vi "VISA MP-285 Get Position Improved Version v070925.vi"(0 "Input: Duty Cluster":T1) -> (1 "Output: X axis (microns)":dbl format="%.2f", 2 "Output: Y axis (microns)":dbl format="%.2f", 3 "Output: Z axis (microns)":dbl format="%.2f", 4 "Output: Duty Cluster":T1)   [LabVIEW 2010]
panel:
  out "Boolean":bool
  out "Serial Read":string
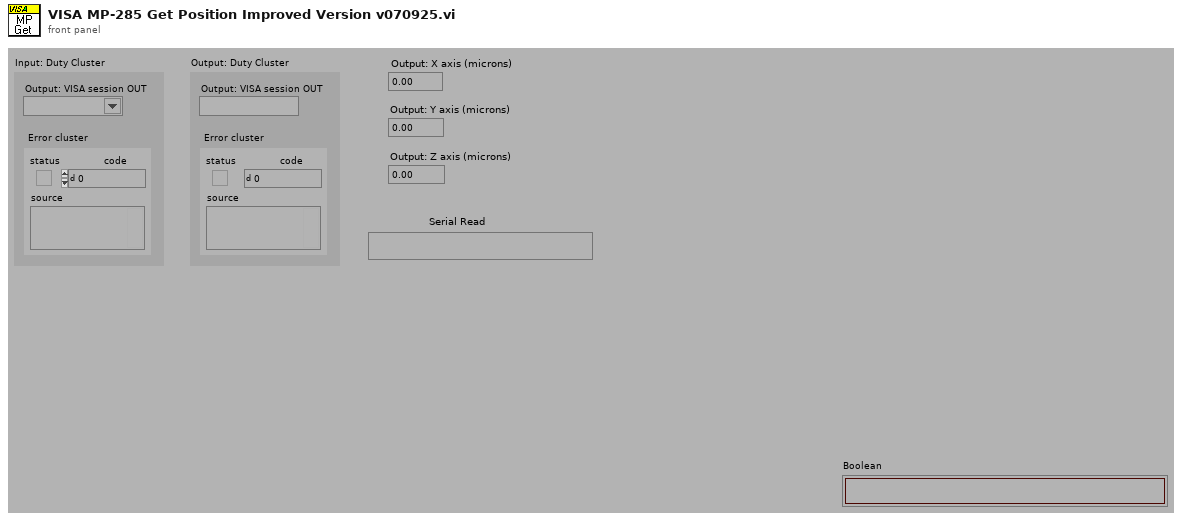
[diagram p1: front panel]
types:
  T1 = cluster{"Output: VISA session OUT":refnum<visa-resource-name>, "Error cluster":errorcluster}
  T2 = cluster{"Output: VISA session OUT":refnum<visa-resource-name>, "error out":errorcluster}
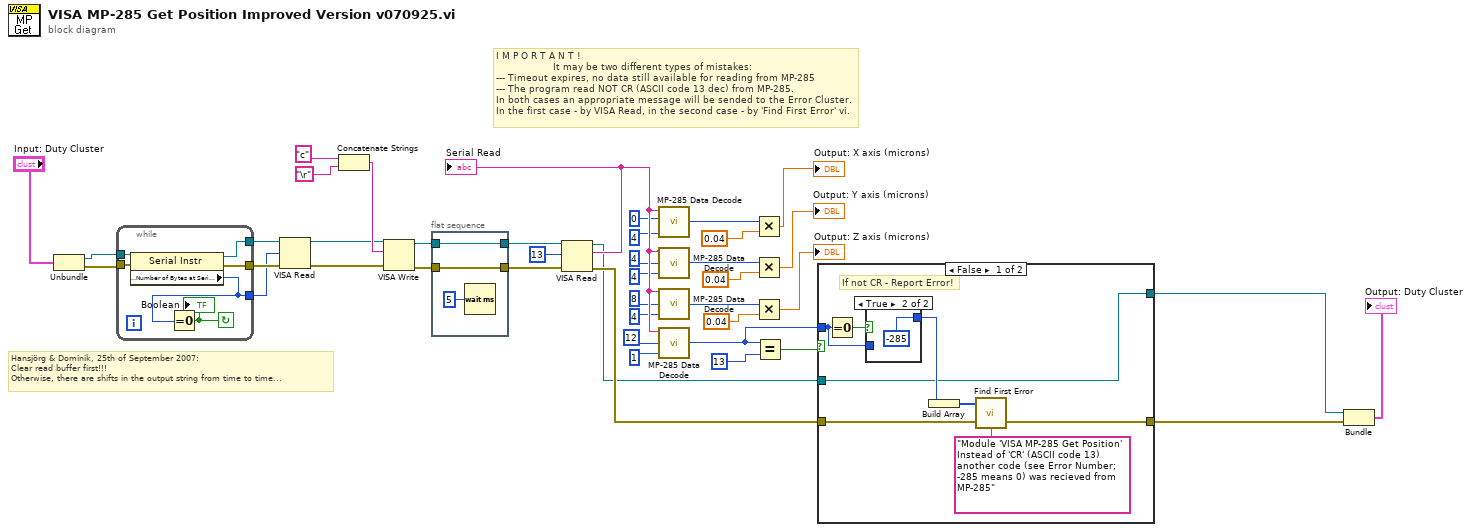
[diagram p0: block diagram]
diagram:
  # "Hansjörg & Dominik, 25th of September 2007: \nClear read buffer first!!!\nOtherwise, there are shifts in the output string from time to time..."
  # "I M P O R T A N T !\n                   It may be two different types of mistakes: \n--- Timeout expires, no data still available for reading from MP-285\n--- The program read NOT CR (ASCII code 13 dec) from MP-285.\nIn both cases an appropriate message will be sended to the Error Cluster.\nIn the first case - by VISA Read, in the second case - by 'Find First Error' vi."
  n1 = Unbundle("Input: Duty Cluster") -> ("Output: VISA session OUT"=w4:refnum<visa-resource-name>, "Error cluster"=w3:errorcluster)
  n2 = while {
    tunnel: [w45] -> w5
    tunnel: [w46] -> w6
    tunnel: [w47] -> w7
    tunnel: w3 -> [w48]
    tunnel: w4 -> [w43]
    stop <- w44 continue-if-true
    n3 = property class="Serial Instr"(reference=w43, error in=w48) -> (reference out=w46:refnum<visa-resource-name>, error out=w47:errorcluster, "Serial Settings:Number of Bytes at Serial Port"=w45:u32)
    n4 = Equal To 0?(x=w45) -> (x = 0?=w44:bool)
    "Boolean" <- w44
  }
  n5 = VISA Read(VISA resource name=w6, byte count=w5, error in (no error)=w7) -> (VISA resource name out=w2:refnum<visa-resource-name>, error out=w1:errorcluster)  [unwired: 2 out]
  n6 = Concatenate Strings("c", "\r") -> (w33:string)
  n7 = VISA Write(VISA resource name=w2, write buffer=w33, error in (no error)=w1) -> (VISA resource name out=w13:refnum<visa-resource-name>, error out=w11:errorcluster)  [unwired: 1 out]
  n8 = flat-sequence {
    tunnel: w13 -> [w51]
    tunnel: [w51] -> w12
    tunnel: w11 -> [w50]
    tunnel: [w50] -> w10
    frame #0 {
      n9 = Wait (ms)(milliseconds to wait=u32 5) -> ()  [unwired: 1 out]
    }
  }
  n10 = VISA Read(VISA resource name=w12, byte count=13, error in (no error)=w10) -> (VISA resource name out=w9:refnum<visa-resource-name>, read buffer=w22:string, error out=w25:errorcluster)  [unwired: 1 out]
  "Serial Read" <- w22
  n11 = call "MP-285 Data Decode.vi"("Input: lenght"=4 ("length"), "Input: offset"=0 ("offset (0)"), "Input: Data string"=w22) -> ("Output: Decoded Data"=w42:i32)
  n12 = call "MP-285 Data Decode.vi"("Input: lenght"=4 ("length"), "Input: offset"=4 ("offset (0)"), "Input: Data string"=w22) -> ("Output: Decoded Data"=w38:i32)
  n13 = call "MP-285 Data Decode.vi"("Input: lenght"=4 ("length"), "Input: offset"=8 ("offset (0)"), "Input: Data string"=w22) -> ("Output: Decoded Data"=w39:i32)
  n14 = call "MP-285 Data Decode.vi"("Input: lenght"=1, "Input: offset"=12, "Input: Data string"=w22) -> ("Output: Decoded Data"=w26:i32)
  n15 = Multiply(x=w42, y=0.04) -> (x*y=→"Output: X axis (microns)":dbl)
  n16 = Multiply(x=w38, y=0.04) -> (x*y=→"Output: Y axis (microns)":dbl)
  n17 = Multiply(x=w39, y=0.04) -> (x*y=→"Output: Z axis (microns)":dbl)
  n18 = Equal?(x=w26, y=13) -> (x = y?=w27:bool)
  n19 = case shown="False" w27 {
    tunnel: [w52 w63] -> w24
    tunnel: w26 -> [w55 _]
    tunnel: w25 -> [w57 w63]
    tunnel: w9 -> [w53 w62]
    tunnel: [w53 w62] -> w8
    frame False {
      # "If not CR - Report Error!"
      n20 = Equal To 0?(x=w55) -> (x = 0?=w56:bool)
      n21 = case shown="True" w56 {
        tunnel: w55 -> [w60 _]
        tunnel: [w60 -285] -> w54
        frame False {
        }
        frame True {
        }
      }
      n22 = Build Array(w54) -> (w58:i32[])
      n23 = call <vilib>:"Find First Error.vi"("error in (no error)"=w57, "source messages"="Module 'VISA MP-285 Get Position'  Instead of 'CR' (ASCII code 13) another code (see Error Number; -285 means 0) was recieved from MP-285", "error codes"=w58) -> ("error out"=w52:errorcluster)  [unwired: 1 in, 1 out]
    }
    frame True {
      # "The CR was readed\n        NO Errors"
      # "TRUE CR was received - NO Errors"
    }
  }
  n24 = Bundle("Output: VISA session OUT"=w8, "error out"=w24) -> (→"Output: Duty Cluster":T2)  [unwired: 1 in]
